vi "resetActiveCycleCounter.vi"(8 "error in (no error)":errorcluster, 11 "Model in":refnum<class "Model.lvclass">) -> (0 "error out":errorcluster, 3 "Model out":refnum<class "Model.lvclass">)   [LabVIEW 2013, in "Model.lvclass"]
uses:
  Model.lvclass
  Model.lvclass/Model.ctl
  ApplicationElements/Log/TestDataLog/TestDataLog.lvclass/TestDataLog.ctl
  UserEvents/UserEvents.lvclass/UserEvents.ctl
  ApplicationElements/TestMonitor/TestMonitor.lvclass
  UserEvents/UserEvents.lvclass
  ApplicationElements/Log/TestDataLog/TestDataLog.lvclass
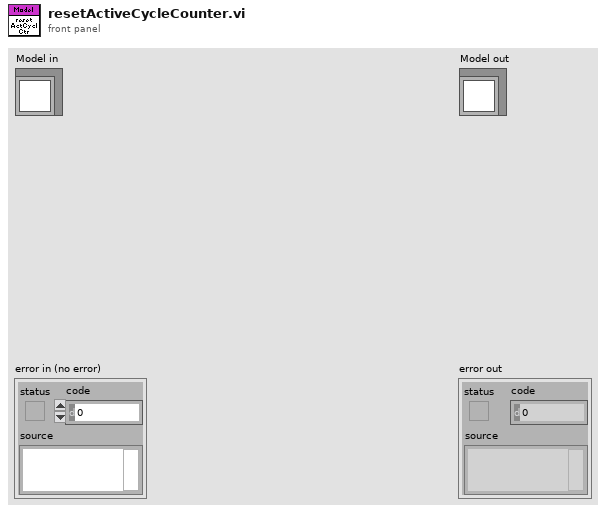
[diagram p1: front panel]
types:
  T1 = typedef "FAMTTypedefs.lvlib/TestStatus.ctl" = cluster{"activeCycle":u32, "activeProfileStep":u32, "demandedCycles":u32, "demandedProfileSteps":u32}
  T2 = typedef "FAMTTypedefs.lvlib/PubDataEvents.ctl" = cluster{"State":refnum<user-event>, "ErrorCode":refnum<user-event>, "OutputData":refnum<user-event>, "InputData":refnum<user-event>, "ControllerData":refnum<user-event>, "TestStatus":refnum<user-event>, "LogPath":refnum<user-event>}
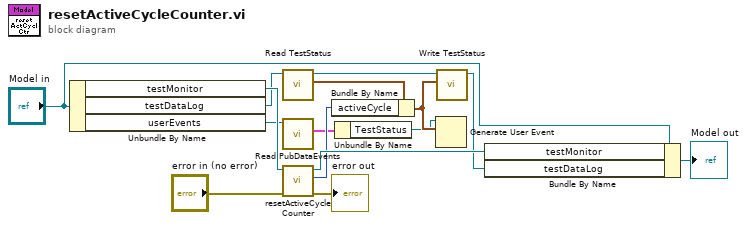
[diagram p0: block diagram]
diagram:
  n1 = Unbundle By Name("Model in") -> ("testMonitor"=w15:refnum<class "TestMonitor.lvclass">, "testDataLog"=w7:refnum<class "TestDataLog.lvclass">, "userEvents"=w1:refnum<class "UserEvents.lvclass">)
  n2 = call "Read TestStatus.vi"("TestDataLog in"=w7) -> ("TestStatus"=w9:T1, "TestDataLog out"=w8:refnum<class "TestDataLog.lvclass">)  [unwired: 9 in]
  n3 = call "Read PubDataEvents.vi"("UserEvents in"=w1) -> ("PubDataEvents"=w3:T2)  [unwired: 9 in, 1 out]
  n4 = call "resetActiveCycleCounter.vi"("error in (no error)"="error in (no error)", "TestMonitor in"=w15) -> ("error out"=→"error out":errorcluster, "activeCycle"=w5:u32, "TestMonitor out"=w12:refnum<class "TestMonitor.lvclass">)  [unwired: 7 in]
  n5 = Bundle By Name(cluster=w9, "activeCycle"=w5) -> (w4:T1)
  n6 = Unbundle By Name(w3) -> ("TestStatus"=w2:refnum<user-event>)
  n7 = Generate User Event(user event=w2, event data cluster=w4) -> ()  [unwired: 2 in, 2 out]
  n8 = call "Write TestStatus.vi"("TestStatus"=w4, "TestDataLog in"=w8) -> ("TestDataLog out"=w6:refnum<class "TestDataLog.lvclass">)  [unwired: 9 in]
  n9 = Bundle By Name(cluster="Model in", "testMonitor"=w12, "testDataLog"=w6) -> (→"Model out":refnum<class "Model.lvclass">)
